vi "File.Rotate.Manager - Reference.vi"() -> (3 "VI Refnum":refnum<vi>)   [LabVIEW 2024, in "EQMF.lvlib" / "File Utils.lvlib" / "File.Rotate.lvclass"]
uses:
  File.Rotate.lvclass
  File.Rotate.Manager - Core.vi
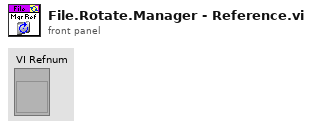
[diagram p1: front panel]
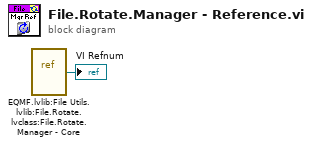
[diagram p0: block diagram]
diagram:
  n1 = vi-ref "EQMF.lvlib:File Utils.lvlib:File.Rotate.lvclass:File.Rotate.Manager - Core.vi"() -> (→"VI Refnum":refnum<vi>)
